vi "check for up_down.vi"(10 "number of zeros numérique":i32=-1, 11 "Array":u16[](array[numeric])) -> (3 "Yes/No":bool)   [LabVIEW 2018]
uses:
  globalVarII.vi
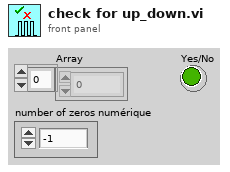
[diagram p1: front panel]
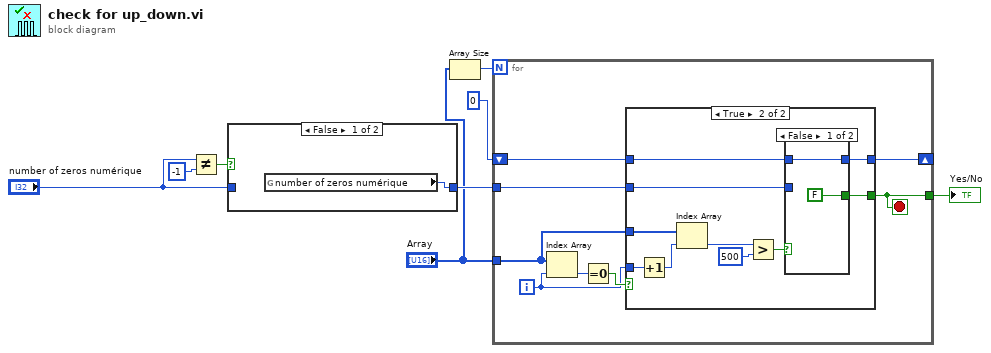
[diagram p0: block diagram]
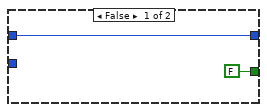
[diagram p3: hidden frame]
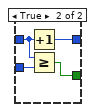
[diagram p4: hidden frame]
diagram:
  n1 = Not Equal?(x="number of zeros numérique", y=-1) -> (x != y?=w5:bool)
  n2 = case shown="False" w5 {
    tunnel: [w9 w10] -> w3
    tunnel: "number of zeros numérique" -> [_ w10]
    frame False {
      n3 = global read "globalVarII.vi" "number of zeros numérique"() -> (w9:i32)
    }
    frame True {
    }
  }
  n4 = Array Size(array="Array") -> (size(s)=w1:i32)
  n5 = for {
    N: w1 -> [_]
    tunnel: "Array" -> [w12]
    shift-right: [w16] -> _
    shift-left: 0 -> [w18]
    tunnel: [w15] -> w7
    tunnel: w3 -> [w14]
    i -> [w11]
    stop <- w15 stop-if-true
    n6 = Index Array(array=w12, index=w11) -> (element=w13:u16)
    n7 = Equal To 0?(x=w13) -> (x = 0?=w17:bool)
    n8 = case shown="True" w17 {
      tunnel: w18 -> [w20 w29]
      tunnel: [w20 w30] -> w16
      tunnel: w14 -> [_ w28]
      tunnel: [FALSE w27] -> w15
      tunnel: w12 -> [_ w26]
      tunnel: w11 -> [_ w25]
      frame False {
      }
      frame True {
        n9 = Increment(x=w25) -> (x+1=w24:i32)
        n10 = Index Array(array=w26, index=w24) -> (element=w23:u16)
        n11 = Greater?(x=w23, y=u16 500) -> (0:w21:bool)
        n12 = case shown="False" w21 {
          tunnel: [w31 w36] -> w30
          tunnel: w29 -> [w31 w35]
          tunnel: w28 -> [_ w34]
          tunnel: [FALSE w33] -> w27
          frame False {
          }
          frame True {
            n13 = Increment(x=w35) -> (x+1=w36:i32)
            n14 = Greater Or Equal?(x=w35, y=w34) -> (x >= y?=w33:bool)
          }
        }
      }
    }
  }
  "Yes/No" <- w7
